vi "Init from Element.vi"(8 "error in (no error)":errorcluster, 10 "Config Element":refnum<class "Config Element.lvclass">, 11 "Condition Config in":refnum<class "Condition Config.lvclass">) -> (0 "error out":errorcluster, 3 "Condition Config out":refnum<class "Condition Config.lvclass">)   [LabVIEW 2020]
uses:
  Condition Config.lvclass
  lv-cdm/CDM-Config/Config Element/Config Element.lvclass
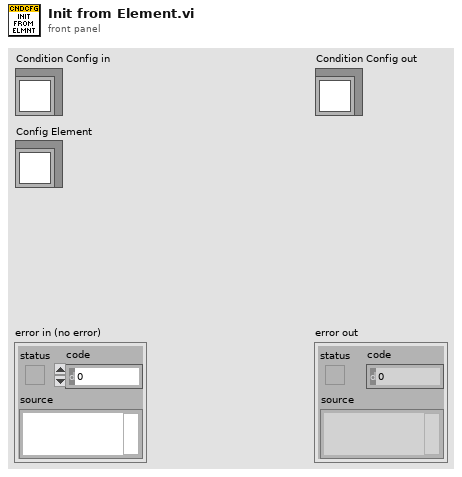
[diagram p1: front panel]
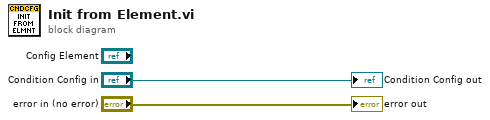
[diagram p0: block diagram]
diagram:
  "error out" <- "error in (no error)"
  "Condition Config out" <- "Condition Config in"
